vi "fgt remove simulated instr.vi"(8 "error in (no error)":errorcluster, 10 "SN":u16, 11 "Type":T1) -> (0 "error out":errorcluster)   [LabVIEW 2016, in "fgt_SDK.lvlib"]
doc: "Removes a simulated instrument that had been previously created. If it had already been initialized by the SDK, the controller and channels will remain in the respective lists, but they will act as if the instrument is missing. This is equivalent to physically disconnecting a real instrument."
uses:
  fgt_SDK.lvlib
  TypeDefs/fgt_INSTRUMENT_TYPE.ctl
  dlls/fgt_SDK_32.dll
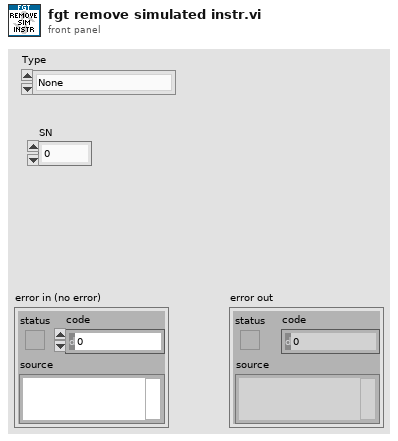
[diagram p1: front panel]
types:
  T1 = typedef "fgt_SDK.lvlib/fgt_INSTRUMENT_TYPE.ctl" = enum32{"None", "MFCS", "MFCS_EZ", "FRP", "LineUP", "IPS"}
  T2 = typedef "fgt_SDK.lvlib/fgt_STATUS_INFO.ctl" = cluster{"InstrType":T1, "instrSN":u16, "errorCode":u8, "infoCode":u8, "detail":string}
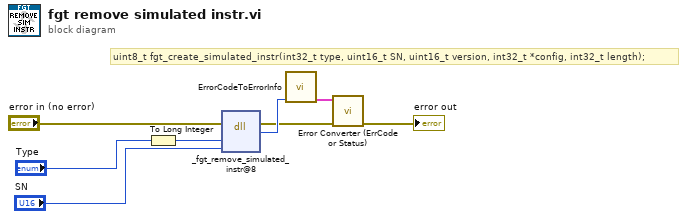
[diagram p0: block diagram]
diagram:
  # "uint8_t fgt_create_simulated_instr(int32_t type, uint16_t SN, uint16_t version, int32_t *config, int32_t length);"
  n1 = To Long Integer(number="Type") -> (32bit integer=w3:i32)
  n2 = dll-call lib="C:/projects/SDK/fgt-sdk-labview/dlls/fgt_SDK_*.*" fn="_fgt_remove_simulated_instr@8"(error in="error in (no error)", "type"=w3, "SN"="SN") -> (error out=w5:errorcluster, "return type"=w6:u8)  [unwired: 4 in, 1 out]
  n3 = call "ErrorCodeToErrorInfo.vi"("return type"=w6) -> ("StatusInfo"=w7:T2)  [unwired: 10 in]
  n4 = call "Error Converter (ErrCode or Status).vi"("error in (no error)"=w5, "StatusInfo"=w7) -> ("error out"=→"error out":errorcluster)  [unwired: 9 in]
